vi "ActivateChnlHW.vi"(8 "error in (no error)":errorcluster, 11 "BME_DG_Chnl in":refnum<class "BME_DG_Chnl.lvclass">) -> (0 "error out":errorcluster, 3 "BME_DG_Chnl out":refnum<class "BME_DG_Chnl.lvclass">)   [LabVIEW 2009, in "BME_DG_Chnl.lvclass"]
uses:
  BME_DG_Chnl.lvclass
  BME_DG_Chnl.lvclass/BME_DG_Chnl.ctl
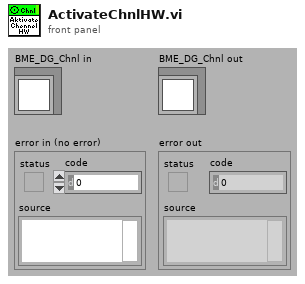
[diagram p1: front panel]
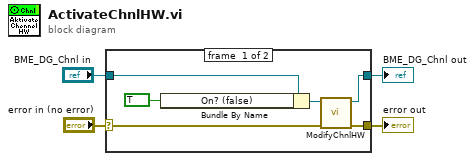
[diagram p0: block diagram]
diagram:
  n1 = case shown="No Error" "error in (no error)" {
    selector: "error in (no error)" -> [w6 w12]
    tunnel: [w5 w12] -> w3
    tunnel: [w7 w11] -> w1
    tunnel: "BME_DG_Chnl in" -> [w10 w11]
    frame #0 {
      n2 = Bundle By Name(cluster=w10, "On? (false)"=TRUE ("ChnParameter.On? (false)")) -> (w8:refnum<class "BME_DG_Chnl.lvclass">)
      n3 = call-dynamic "ModifyChnlHW.vi"("error in (no error)"=w6, "BME_DG_Chnl in"=w8) -> ("error out"=w5:errorcluster, "BME_DG_Chnl out"=w7:refnum<class "BME_DG_Chnl.lvclass">)  [unwired: 8 in]
    }
    frame #1 {
    }
  }
  "error out" <- w3
  "BME_DG_Chnl out" <- w1
